vi "VisualizationManager.vi"(7 "Action":T1, 8 "error in (no error)":errorcluster, 9 "Load In SubPanel?":bool, 10 "Module Name":string, 11 "Open Visualization VIs in":T2[](array[typedef])) -> (0 "error out":errorcluster, 1 "In SubPanel?":bool, 2 "Module Name out":string, 3 "Open Visualization VIs out":T2[](array[typedef]))   [LabVIEW 2018]
uses:
  OpenVisualizationVIs.ctl
  VisualizationManagerActions.ctl
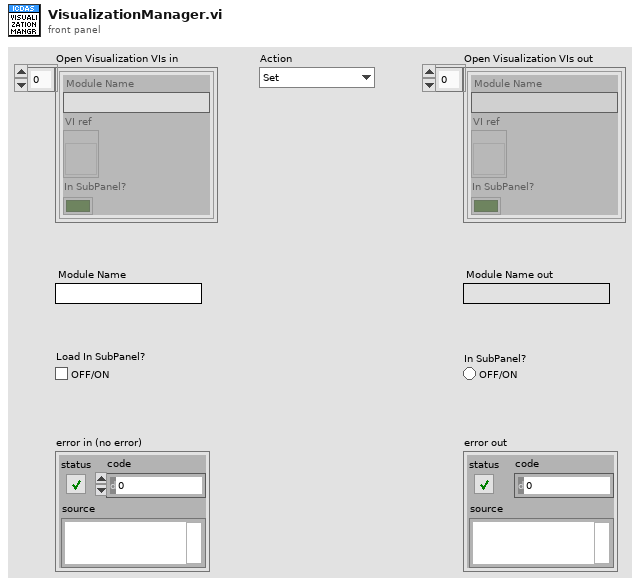
[diagram p1: front panel]
types:
  T1 = typedef "VisualizationManagerActions.ctl" = enum16{"Set", "LoadModVI", "PopInOutModVI", "Add", "Clear"}
  T2 = typedef "OpenVisualizationVIs.ctl" = cluster{"Module Name":string, "VI ref":refnum<vi>, "In SubPanel?":bool}
  T3 = enum32{"Invalid", "Standard", "Closed", "Hidden", "Minimized", "Maximized"}
  T4 = typedef "cntlRefs.ctl" = cluster{"rngFGen":refnum<vi>, "rngDigitizer":refnum<vi>, "btnHide":refnum<vi>, "rngInst":refnum<vi>, "Instrument Modules":refnum<vi>, "RelativePathToINIFiles ":refnum<vi>, "PluginTree":refnum<vi>, "TestTree":refnum<vi>, "path.tstFile":refnum<vi>, "cmbxRunningModules":refnum<vi>, "TestDataSubPanel":refnum<vi>, "TestDataCaption":refnum<vi>, "btnPopInOut":refnum<vi>}
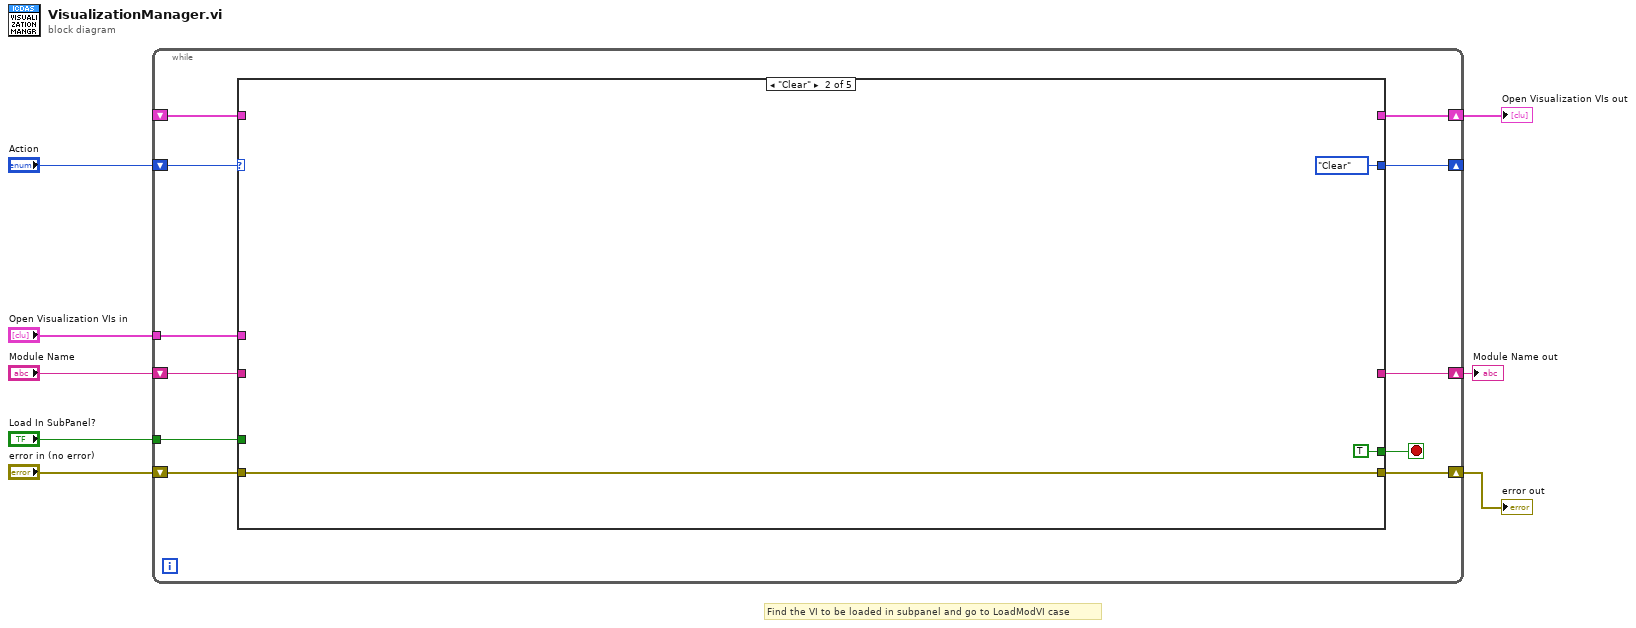
[diagram p0: block diagram]
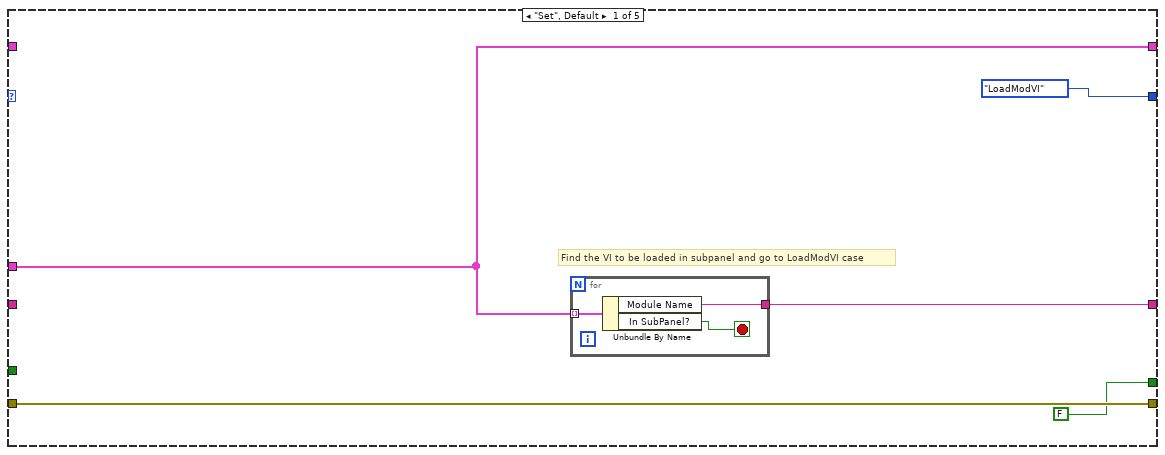
[diagram p2: hidden frame]
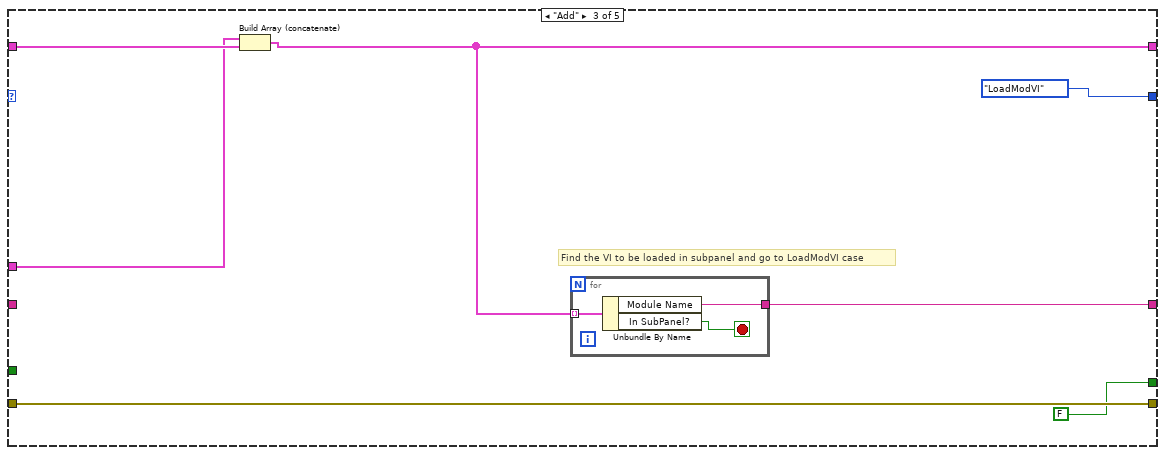
[diagram p3: hidden frame]
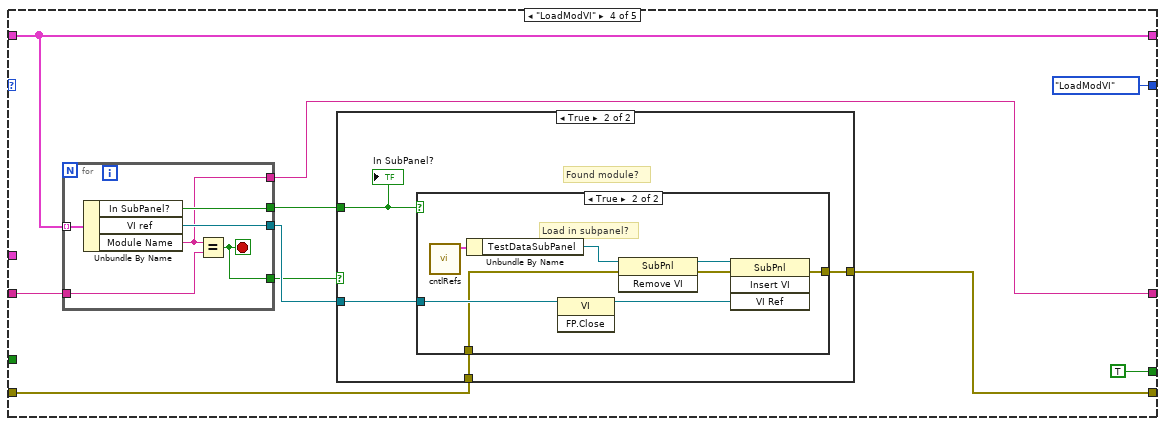
[diagram p4: hidden frame]
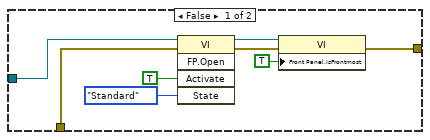
[diagram p6: hidden frame]
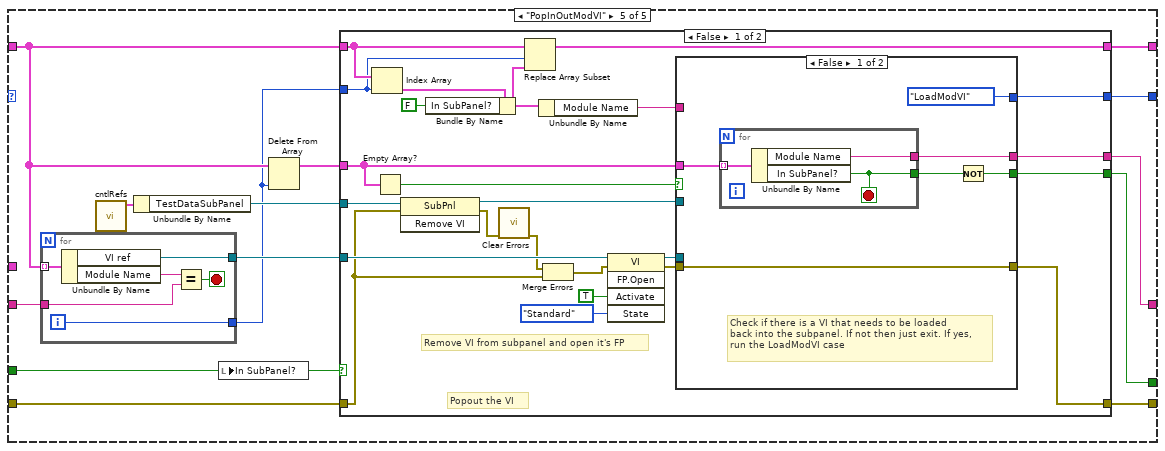
[diagram p7: hidden frame]
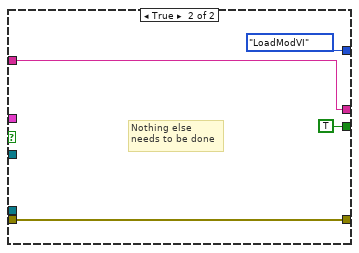
[diagram p8: hidden frame]
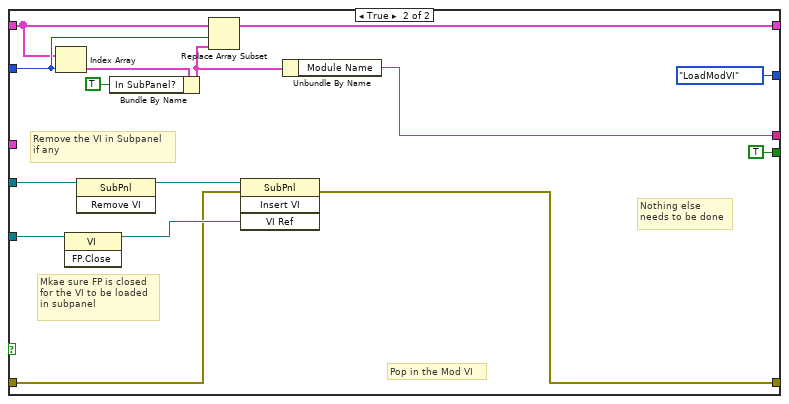
[diagram p9: hidden frame]
diagram:
  # "Find the VI to be loaded in subpanel and go to LoadModVI case"
  n1 = while {
    tunnel: "Load In SubPanel?" -> [w13]
    shift-right: [w19] -> w8
    shift-left: "error in (no error)" -> [w18]
    tunnel: "Open Visualization VIs in" -> [w16]
    shift-right: [w15] -> w4
    shift-left: _ -> [w11]
    shift-right: [w10] -> _
    shift-left: "Action" -> [w14]
    shift-right: [w9] -> w1
    shift-left: "Module Name" -> [w17]
    stop <- w12 stop-if-true
    n2 = case shown="\"Clear\"" w14 {
      tunnel: w16 -> [w22 _ w31 _ _]
      tunnel: [w22 _ w32 w47 w78] -> w15
      tunnel: w11 -> [_ _ w33 w47 w80]
      tunnel: w17 -> [_ _ _ w50 w86]
      tunnel: w18 -> [w24 w30 w37 w48 w87]
      tunnel: [w24 w30 w37 w46 w88] -> w19
      tunnel: w13 -> [_ _ _ _ w77]
      tunnel: [FALSE TRUE FALSE TRUE w82] -> w12
      tunnel: [VisualizationManagerActions."LoadModVI" ("Action") VisualizationManagerActions."Clear" ("Action") VisualizationManagerActions."LoadModVI" ("Action") VisualizationManagerActions."LoadModVI" ("Action") w83] -> w10
      tunnel: [w21 _ w35 w41 w81] -> w9
      frame "Set", Default {
        # "Find the VI to be loaded in subpanel and go to LoadModVI case"
        n3 = for {
          tunnel: w22 -> [w27] mode=indexing
          tunnel: [w26] -> w21
          stop <- w25 stop-if-true
          n4 = Unbundle By Name(w27) -> ("Module Name"=w26:string, "In SubPanel?"=w25:bool)
        }
      }
      frame "Clear" {
      }
      frame "Add" {
        # "Find the VI to be loaded in subpanel and go to LoadModVI case"
        n5 = Build Array (concatenate)(w31, w33) -> (w32:T2[])
        n6 = for {
          tunnel: w32 -> [w40] mode=indexing
          tunnel: [w39] -> w35
          stop <- w38 stop-if-true
          n7 = Unbundle By Name(w40) -> ("Module Name"=w39:string, "In SubPanel?"=w38:bool)
        }
      }
      frame "LoadModVI" {
        n8 = for {
          tunnel: w47 -> [w76] mode=indexing
          tunnel: w50 -> [w75]
          tunnel: [w74] -> w49
          tunnel: [w73] -> w45
          tunnel: [w72] -> w44
          tunnel: [w71] -> w41
          stop <- w73 stop-if-true
          n9 = Unbundle By Name(w76) -> ("In SubPanel?"=w72:bool, "VI ref"=w74:refnum<vi>, "Module Name"=w71:string)
          n10 = Equal?(x=w71, y=w75) -> (x = y?=w73:bool)
        }
        n11 = case shown="True" w45 {
          tunnel: w49 -> [_ w55]
          tunnel: w48 -> [w51 w54]
          tunnel: [w51 w53] -> w46
          tunnel: w44 -> [_ w52]
          frame False {
          }
          frame True {
            # "Found module?"
            n12 = case shown="True" w52 {
              tunnel: w55 -> [w61 w70]
              tunnel: w54 -> [w60 w69]
              tunnel: [w58 w68] -> w53
              frame False {
                n13 = invoke class="VI" method="FP.Open"(reference=w61, error in=w60, "Activate"=TRUE ("Activate?"), "State"=T3."Standard") -> (reference out=w57:refnum<vi>, error out=w59:errorcluster)  [unwired: 1 in, 3 out]
                n14 = property class="VI"(reference=w57, error in=w59, "Front Panel.IsFrontmost"=TRUE ("Front Panel Window:Is Frontmost")) -> (error out=w58:errorcluster)  [unwired: 1 out]
              }
              frame True {
                # "Load in subpanel?"
                n15 = call "cntlRefs.vi"() -> ("cntlRefs"=w66:T4)  [unwired: 10 in, 1 out]
                n16 = Unbundle By Name(w66) -> ("TestDataSubPanel"=w64:refnum<vi>)
                n17 = invoke class="VI" method="FP.Close"(reference=w70) -> (reference out=w65:refnum<vi>)  [unwired: 2 in, 2 out]
                n18 = invoke class="SubPnl" method="Remove VI"(reference=w64) -> (reference out=w67:refnum<vi>)  [unwired: 2 in, 2 out]
                n19 = invoke class="SubPnl" method="Insert VI"(reference=w67, error in=w69, "VI Ref"=w65) -> (error out=w68:errorcluster)  [unwired: 1 in, 3 out]
              }
            }
            "In SubPanel?" <- w52
          }
        }
      }
      frame "PopInOutModVI" {
        n20 = for {
          tunnel: w80 -> [w148] mode=indexing
          tunnel: w86 -> [w146]
          tunnel: [w144] -> w85
          tunnel: [w143] -> w79
          i -> [w143]
          stop <- w145 stop-if-true
          n21 = Unbundle By Name(w148) -> ("VI ref"=w144:refnum<vi>, "Module Name"=w147:string)
          n22 = Equal?(x=w147, y=w146) -> (x = y?=w145:bool)
        }
        n23 = call "cntlRefs.vi"() -> ("cntlRefs"=w89:T4)  [unwired: 10 in, 1 out]
        n24 = Unbundle By Name(w89) -> ("TestDataSubPanel"=w90:refnum<vi>)
        n25 = local write "In SubPanel?"(w77) -> ()
        n26 = Delete From Array(array=w80, index=w79) -> (array with subset deleted=w84:T2[])  [unwired: 1 in, 1 out]
        n27 = case shown="False" w77 {
          tunnel: w90 -> [w114 w142]
          tunnel: [w100 w130] -> w88
          tunnel: w87 -> [w103 w133]
          tunnel: w85 -> [w111 w136]
          tunnel: w84 -> [w109 _]
          tunnel: [w101 VisualizationManagerActions."LoadModVI" ("Action")] -> w83
          tunnel: [w99 TRUE] -> w82
          tunnel: [w98 w128] -> w81
          tunnel: w80 -> [w97 w138]
          tunnel: w79 -> [w94 w139]
          tunnel: [w96 w137] -> w78
          frame False {
            # "Remove VI from subpanel and open it's FP"
            # "Popout the VI"
            n28 = Index Array(array=w97, index=w94) -> (element=w95:T2)
            n29 = Empty Array?(array=w109) -> (empty?=w110:bool)
            n30 = invoke class="SubPnl" method="Remove VI"(reference=w114, error in=w103) -> (reference out=w106:refnum<vi>, error out=w105:errorcluster)  [unwired: 1 in, 1 out]
            n31 = Bundle By Name(cluster=w95, "In SubPanel?"=FALSE) -> (w92:T2)
            n32 = call <vilib>:"Clear Errors.vi"("error in (no error)"=w105) -> ("error out"=w104:errorcluster)  [unwired: 5 in, 1 out]
            n33 = Replace Array Subset(array=w97, new element=w92, index=w94) -> (w96:T2[])
            n34 = Unbundle By Name(w92) -> ("Module Name"=w91:string)
            n35 = Merge Errors(w104, w103) -> (w102:errorcluster)
            n36 = invoke class="VI" method="FP.Open"(reference=w111, error in=w102, "Activate"=TRUE ("Activate?"), "State"=T3."Standard") -> (reference out=w107:refnum<vi>, error out=w108:errorcluster)  [unwired: 1 in, 3 out]
            n37 = case shown="False" w110 {
              tunnel: w109 -> [w119 _]
              tunnel: w108 -> [w118 w127]
              tunnel: w107 -> [_ _]
              tunnel: w106 -> [_ _]
              tunnel: [VisualizationManagerActions."LoadModVI" ("Action") VisualizationManagerActions."LoadModVI" ("Action")] -> w101
              tunnel: [w118 w127] -> w100
              tunnel: [w116 TRUE] -> w99
              tunnel: [w115 w124] -> w98
              tunnel: w91 -> [_ w124]
              frame False {
                # "Check if there is a VI that needs to be loaded\nback into the subpanel. If not then just exit. If yes,\nrun the LoadModVI case"
                n38 = for {
                  tunnel: w119 -> [w123] mode=indexing
                  tunnel: [w122] -> w115
                  tunnel: [w121] -> w117
                  stop <- w121 stop-if-true
                  n39 = Unbundle By Name(w123) -> ("Module Name"=w122:string, "In SubPanel?"=w121:bool)
                }
                n40 = Not(x=w117) -> (.not. x?=w116:bool)
              }
              frame True {
                # "Nothing else\nneeds to be done"
              }
            }
          }
          frame True {
            # "Nothing else\nneeds to be done"
            # "Mkae sure FP is closed\nfor the VI to be loaded\nin subpanel"
            # "Remove the VI in Subpanel\nif any"
            # "Pop in the Mod VI"
            n41 = Index Array(array=w138, index=w139) -> (element=w141:T2)
            n42 = invoke class="VI" method="FP.Close"(reference=w136) -> (reference out=w134:refnum<vi>)  [unwired: 2 in, 2 out]
            n43 = invoke class="SubPnl" method="Remove VI"(reference=w142) -> (reference out=w135:refnum<vi>)  [unwired: 2 in, 2 out]
            n44 = Bundle By Name(cluster=w141, "In SubPanel?"=TRUE) -> (w129:T2)
            n45 = Replace Array Subset(array=w138, new element=w129, index=w139) -> (w137:T2[])
            n46 = invoke class="SubPnl" method="Insert VI"(reference=w135, error in=w133, "VI Ref"=w134) -> (error out=w130:errorcluster)  [unwired: 1 in, 3 out]
            n47 = Unbundle By Name(w129) -> ("Module Name"=w128:string)
          }
        }
      }
    }
  }
  "error out" <- w8
  "Open Visualization VIs out" <- w4
  "Module Name out" <- w1
